vi "getState.vi"(8 "error in (no error)":errorcluster, 11 "State in":refnum<class "ReadingBufferState.lvclass">) -> (0 "error out":errorcluster, 2 "StateValue":T1=enum."DisabledState", 3 "State out":refnum<class "ReadingBufferState.lvclass">)   [LabVIEW 2016, in "ReadingBufferState.lvclass"]
uses:
  ReadingBufferState.lvclass
  ts_electrometeruserevents/Typedefs/StateValue.ctl
  ts_electrometeruserevents/Typedefs/ElectrometerTypedefs.lvlib
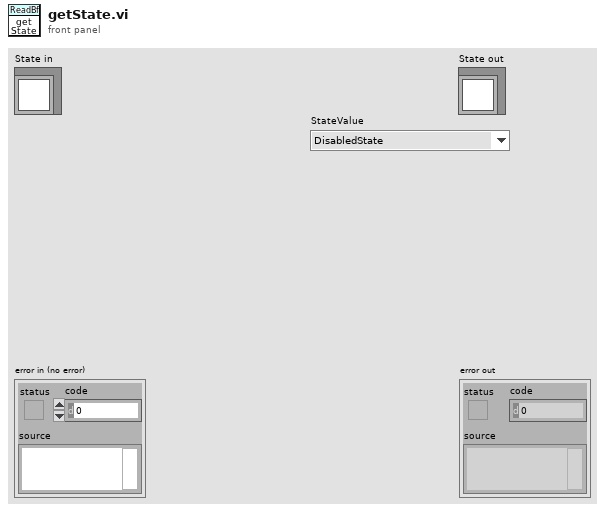
[diagram p1: front panel]
types:
  T1 = typedef "ElectrometerTypedefs.lvlib/StateValue.ctl" = enum16{"", "DisabledState", "EnabledState", "FaultState", "OffState", "StandbyState", "ReadyState", "ConfiguringState", "ManualReadingState", "UntilIntensityReadingState", "SetDurationReadingState", "BufferReadingState"}
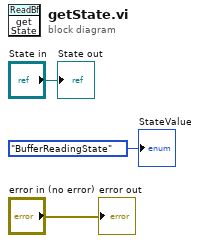
[diagram p0: block diagram]
diagram:
  "error out" <- "error in (no error)"
  "State out" <- "State in"
  "StateValue" <- StateValue."BufferReadingState" ("StateValue")
